vi "Keithley 6517A System Functions.vi"(0 "GPIB address":string="27", 1 "Hours":i16=12 min=0 max=23 step=1, 2 "Minutes":i16 min=0 max=59 step=1, 3 "Seconds":i16 min=0 max=59 step=1, 4 "Line-Sync":bool, 5 "System Functions":u16(ring) items=["Reset Reading Number", "Reset Relative Timestamp", "Save Configuration", "Recall Configuration", "Set Power-On State", "Line-Sync Controls", "Set Time and Date", "Select Timestamp Type", "External Temperature Control", "A/D Hardware Limit Control", "Humidity Reading Control"], 6 "External Temperature":bool, 7 "Save, Recall, or Power-on Selection":i16(knob) min=0 max=11 step=1 scale=0.0..11.0, 8 "A/D Hardware Limit Control":bool=TRUE, 9 "TimeStamp Type":u16(ring) items=["Relative", "Real"], 10 "Humidity Reading Control":bool, 11 "error in":T1, 12 "Year":i16=1998 min=1998 max=2092 step=1, 13 "Month":i16=1 min=1 max=12 step=1, 14 "Day":i16=1 min=1 max=31 step=1) -> (15 "error out":T1)   [LabVIEW 2024]
doc: "This VI is used to perform some of the basic system commands such as setting the Real-Time clock, setting power-on settings, controlling line-sync, external temperature, A/D limits, and humidity functions. These commands are optional and do not need to be performed for any specified type of measurement.\n\nSystem Functions:\n0 = Reset Reading Number\n1 = Reset Relative Timestamp\n2 = Save Configuration\n3 = Recall Configuration\n4 = Set Power-On State\n5 = Line-Sync Controls\n6 = Set Time and Date\n7 = Select Time Stamp Type\n8 = External Temperature Control\n9 = A/D Hardware Limit Control\n10 = Humidity Reading Control\n\nLine-Sync:\nTrue = On\nFalse = Off\n\nExternal Temperature\nTrue = On\nFalse = Off\n\nA/D Hardware Limit\nTrue = On\nFalse = Off\n\nHumidity Reading Control\nTrue = On\nFalse = Off\n\nSave, Recall, or Power-on Selection\n0 = SAV0\n1 = SAV1\n2 = SAV2\n3 = SAV3\n4 = SAV4\n5 = SAV5\n6 = SAV6\n7 = SAV7\n8 = SAV8\n9 = SAV9\n10 = RST\n11 = PRESET\n\nTimeStamp Type:\n0 = Relative\n1 = Real"
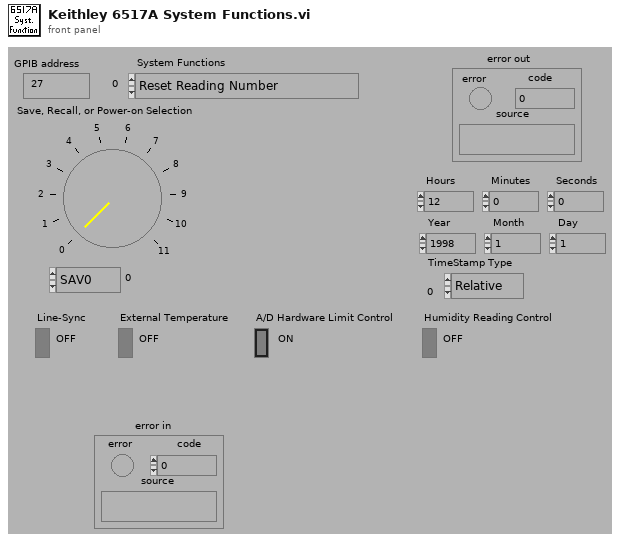
[diagram p1: front panel]
types:
  T1 = cluster{"error":bool, "code":i32, "source":string}
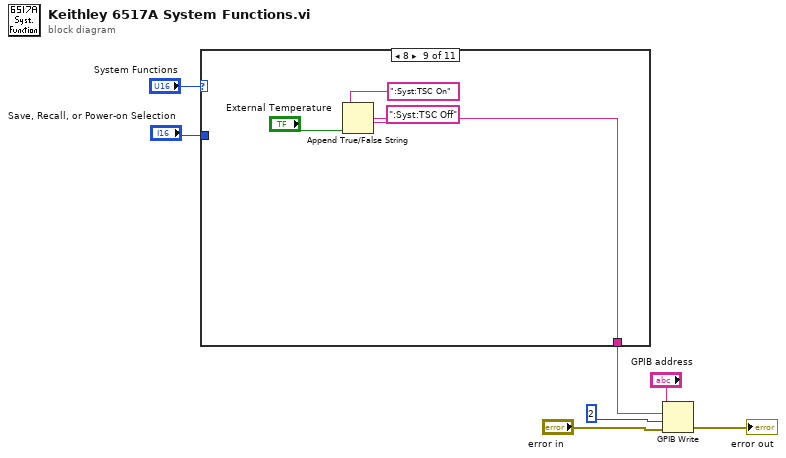
[diagram p0: block diagram]
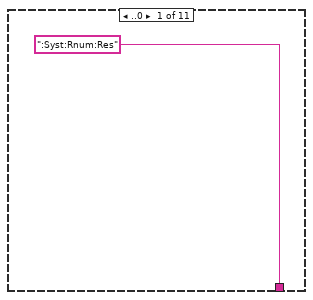
[diagram p2: hidden frame]
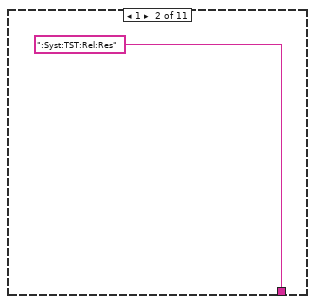
[diagram p3: hidden frame]
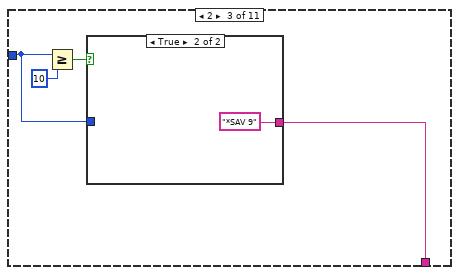
[diagram p4: hidden frame]
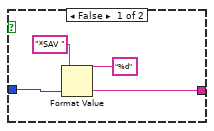
[diagram p5: hidden frame]
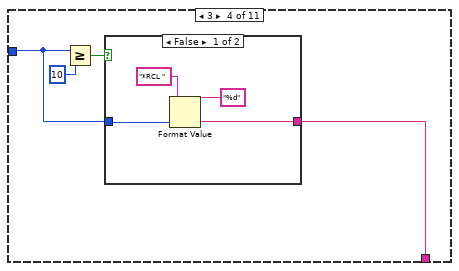
[diagram p6: hidden frame]
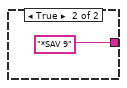
[diagram p7: hidden frame]
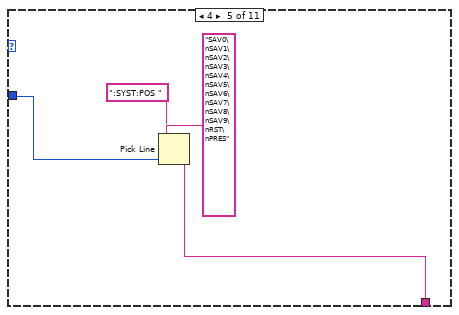
[diagram p8: hidden frame]
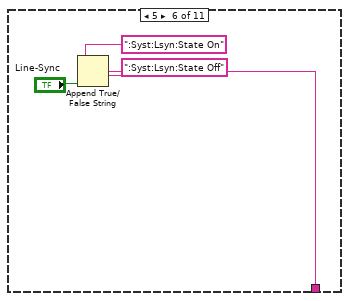
[diagram p9: hidden frame]
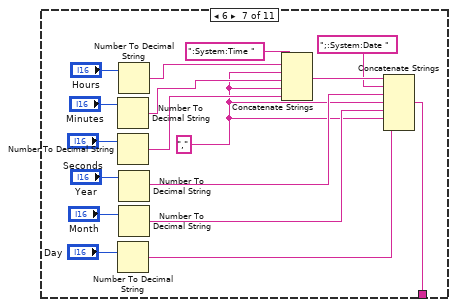
[diagram p10: hidden frame]
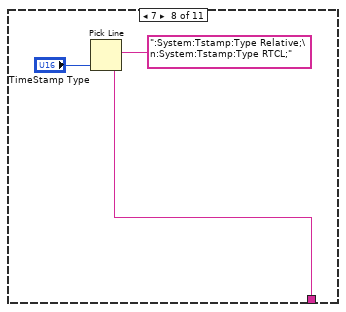
[diagram p11: hidden frame]
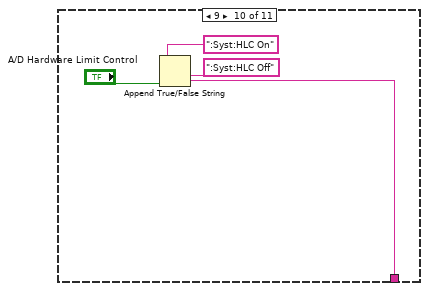
[diagram p12: hidden frame]
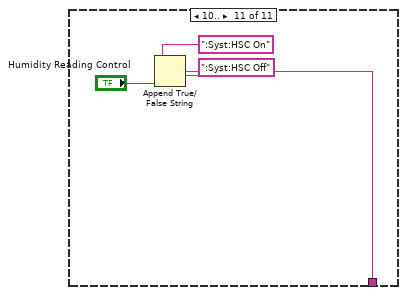
[diagram p13: hidden frame]
diagram:
  n1 = case shown="8" "System Functions" {
    tunnel: "Save, Recall, or Power-on Selection" -> [_ _ w10 w20 w29 _ _ _ _ _ _]
    tunnel: [":Syst:Rnum:Res" ":Syst:TST:Rel:Res" w11 w19 w28 w32 w41 w53 w56 w60 w64] -> w1
    frame ..0 {
    }
    frame 1 {
    }
    frame 2 {
      n2 = Greater Or Equal?(x=w10, y=10) -> (x >= y?=w12:bool)
      n3 = case shown="True" w12 {
        tunnel: [w15 "*SAV 9"] -> w11
        tunnel: w10 -> [w14 _]
        frame False {
          n4 = Format Value(string ("")="*SAV ", format string="%d", value (0)=w14) -> (output string=w15:string)
        }
        frame True {
        }
      }
    }
    frame 3 {
      n5 = Greater Or Equal?(x=w20, y=10) -> (x >= y?=w21:bool)
      n6 = case shown="False" w21 {
        tunnel: w20 -> [w24 _]
        tunnel: [w23 "*SAV 9"] -> w19
        frame False {
          n7 = Format Value(string ("")="*RCL ", format string="%d", value (0)=w24) -> (output string=w23:string)
        }
        frame True {
        }
      }
    }
    frame 4 {
      n8 = Pick Line(string ("")=":SYST:POS ", multi-line string="SAV0\nSAV1\nSAV2\nSAV3\nSAV4\nSAV5\nSAV6\nSAV7\nSAV8\nSAV9\nRST\nPRES", line index=w29) -> (output string=w28:string)
    }
    frame 5 {
      n9 = Append True/False String(1:"Line-Sync", 2:":Syst:Lsyn:State Off", 3:":Syst:Lsyn:State On") -> (0:w32:string)  [unwired: 1 in]
    }
    frame 6 {
      w36 = ","
      n10 = Number To Decimal String(number="Minutes") -> (decimal integer string=w39:string)  [unwired: 1 in]
      n11 = Number To Decimal String(number="Seconds") -> (decimal integer string=w37:string)  [unwired: 1 in]
      n12 = Number To Decimal String(number="Day") -> (decimal integer string=w51:string)  [unwired: 1 in]
      n13 = Number To Decimal String(number="Hours") -> (decimal integer string=w38:string)  [unwired: 1 in]
      n14 = Number To Decimal String(number="Year") -> (decimal integer string=w49:string)  [unwired: 1 in]
      n15 = Number To Decimal String(number="Month") -> (decimal integer string=w50:string)  [unwired: 1 in]
      n16 = Concatenate Strings(":System:Time ", w38, w36, w39, w36, w37) -> (w52:string)
      n17 = Concatenate Strings(w52, ";:System:Date ", w49, w36, w50, w36, w51) -> (w41:string)
    }
    frame 7 {
      n18 = Pick Line(multi-line string=":System:Tstamp:Type Relative;\n:System:Tstamp:Type RTCL;", line index="TimeStamp Type") -> (output string=w53:string)  [unwired: 1 in]
    }
    frame 8 {
      n19 = Append True/False String(1:"External Temperature", 2:":Syst:TSC Off", 3:":Syst:TSC On") -> (0:w56:string)  [unwired: 1 in]
    }
    frame 9 {
      n20 = Append True/False String(1:"A/D Hardware Limit Control", 2:":Syst:HLC Off", 3:":Syst:HLC On") -> (0:w60:string)  [unwired: 1 in]
    }
    frame 10.. {
      n21 = Append True/False String(1:"Humidity Reading Control", 2:":Syst:HSC Off", 3:":Syst:HSC On") -> (0:w64:string)  [unwired: 1 in]
    }
  }
  n22 = GPIB Write(0:"GPIB address", 1:w1, 2:2, 3:"error in") -> (6:→"error out":errorcluster)  [unwired: 1 in, 1 out]
